vi "AbortGeneration.vi"(8 "error in (no error)":errorcluster, 11 "DaqMx_Single in":refnum<class "DaqMx_Single.lvclass">) -> (0 "error out":errorcluster, 3 "DaqMx_Single out":refnum<class "DaqMx_Single.lvclass">)   [LabVIEW 2014, in "FgenPlugins.lvlib" / "DaqMx_Single.lvclass"]
uses:
  DaqMx_Single.lvclass
  NiPxi6733Class/NiPxi6733.lvclass
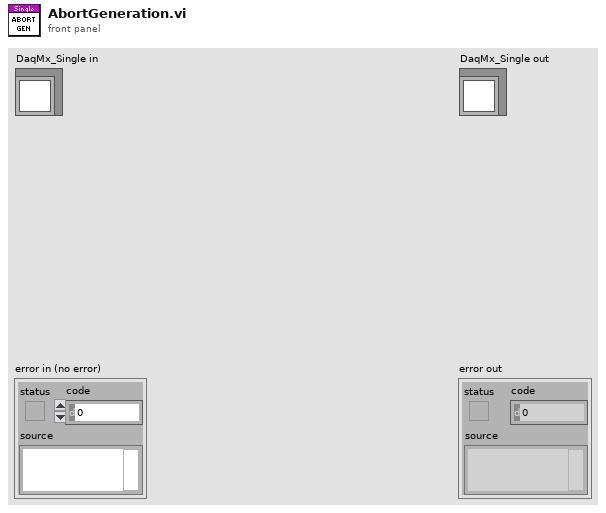
[diagram p1: front panel]
types:
  T1 = typedef "FgenPlugins.lvlib/DaqMx_Single.lvclass/clEvents.ctl" = cluster{"Stop":refnum<user-event>, "Params":refnum<user-event>}
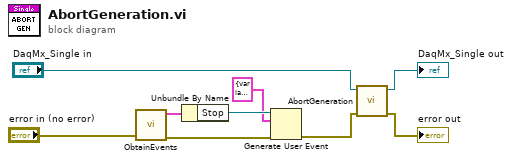
[diagram p0: block diagram]
diagram:
  n1 = call "ObtainEvents.vi"("error in (no error)"="error in (no error)") -> ("error out"=w5:errorcluster, "clEvent"=w8:T1)  [unwired: 9 in]
  n2 = Unbundle By Name(w8) -> ("Stop"=w7:refnum<user-event>)
  n3 = Generate User Event(user event=w7, event data cluster=cluster{"Data":variant} {"Data"=variant} ("event data"), error in=w5) -> (error out=w3:errorcluster)  [unwired: 1 in, 1 out]
  n4 = call-parent "AbortGeneration.vi"("error in (no error)"=w3, "NiPxi6733 in"="DaqMx_Single in") -> ("error out"=→"error out":errorcluster, "NiPxi6733 out"=→"DaqMx_Single out":refnum<class "DaqMx_Single.lvclass">)  [unwired: 8 in]
